vi "Variant To String.vi"(7 "Unsupported (Empty)":string, 10 "Variant":variant) -> (2 "Supported":bool, 3 "String":string)   [LabVIEW 2020, in "FlexBlocks.lvlib"]
uses:
  FlexBlocks.lvlib
  <vilib>/Utility/Data Type/NI_Data Type.lvlib
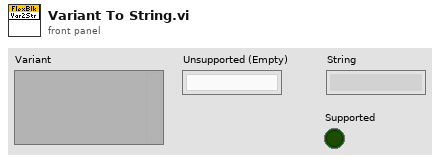
[diagram p1: front panel]
types:
  T1 = typedef "NI_Data Type.lvlib/Data Type.ctl" = enum8{"Invalid Type", "Void", "I8", "I16", "I32", "I64", "U8", "U16", "U32", "U64", "Single Float", "Double Float", "Extended Float", "Single Complex", "Double Complex", "Extended Complex", "Enum U8", "Enum U16", "Enum U32", "Enum U64", "Single Float With Unit", "Double Float With Unit", "Extended Float With Unit", "Single Complex with Unit", "Double Complex with Unit", "Extended Complex with Unit", "Boolean", "String", "Path", "Picture", "Tag", "Array", "Cluster", "Variant", "LV Variant", "Waveform", "Timestamp", "Digital Waveform", "Digital Data", "ExpressData", "Refnum", "External Data", "VI", "Poly VI", "LabVIEW Class Instance", "Fixed Point", "Set Collection", "Map Collection"}
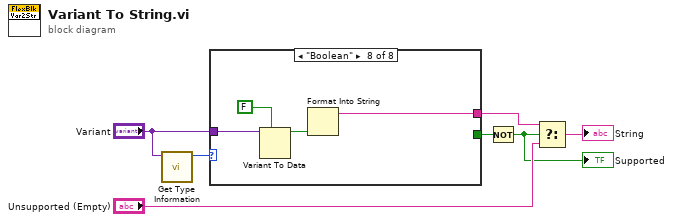
[diagram p0: block diagram]
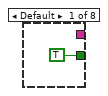
[diagram p2: hidden frame]
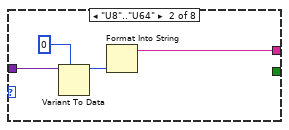
[diagram p3: hidden frame]
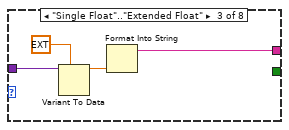
[diagram p4: hidden frame]
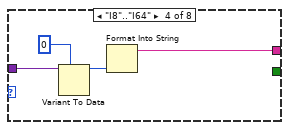
[diagram p5: hidden frame]
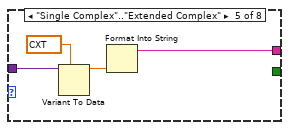
[diagram p6: hidden frame]
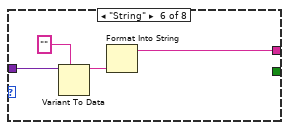
[diagram p7: hidden frame]
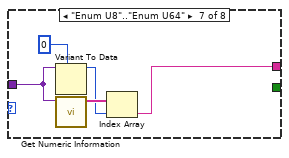
[diagram p8: hidden frame]
diagram:
  n1 = call <vilib>:"Get Type Information.vi"("variant"="Variant") -> ("type"=w5:T1)  [unwired: 6 in, 4 out]
  n2 = case shown="\"Boolean\"" w5 {
    tunnel: [TRUE _ _ _ _ _ _ _] -> w4
    tunnel: "Variant" -> [_ w12 w16 w20 w24 w28 w33 w37]
    tunnel: [_ w9 w13 w17 w21 w25 w29 w34] -> w1
    frame Default {
    }
    frame "U8".."U64" {
      n3 = Variant To Data(type=u64 0 ("U64"), Variant=w12) -> (data=w10:u64)  [unwired: 1 in, 1 out]
      n4 = Format Into String(w10) -> (resulting string=w9:string)  [unwired: 3 in, 1 out]
    }
    frame "Single Float".."Extended Float" {
      n5 = Variant To Data(type=ext 0.0 ("Ext"), Variant=w16) -> (data=w14:ext)  [unwired: 1 in, 1 out]
      n6 = Format Into String(w14) -> (resulting string=w13:string)  [unwired: 3 in, 1 out]
    }
    frame "I8".."I64" {
      n7 = Variant To Data(type=i64 0 ("I64"), Variant=w20) -> (data=w18:i64)  [unwired: 1 in, 1 out]
      n8 = Format Into String(w18) -> (resulting string=w17:string)  [unwired: 3 in, 1 out]
    }
    frame "Single Complex".."Extended Complex" {
      n9 = Variant To Data(type=cxt 0.0+0.0i ("I64"), Variant=w24) -> (data=w22:cxt)  [unwired: 1 in, 1 out]
      n10 = Format Into String(w22) -> (resulting string=w21:string)  [unwired: 3 in, 1 out]
    }
    frame "String" {
      n11 = Variant To Data(type="" ("I64"), Variant=w28) -> (data=w26:string)  [unwired: 1 in, 1 out]
      n12 = Format Into String(w26) -> (resulting string=w25:string)  [unwired: 3 in, 1 out]
    }
    frame "Enum U8".."Enum U64" {
      n13 = Variant To Data(type=u64 0, Variant=w33) -> (data=w30:u64)  [unwired: 1 in, 1 out]
      n14 = call <vilib>:"Get Numeric Information.vi"("variant"=w33) -> ("enum names"=w31:string[])  [unwired: 7 in, 3 out]
      n15 = Index Array(array=w31, index=w30) -> (element=w29:string)
    }
    frame "Boolean" {
      n16 = Variant To Data(type=FALSE, Variant=w37) -> (data=w35:bool)  [unwired: 1 in, 1 out]
      n17 = Format Into String(w35) -> (resulting string=w34:string)  [unwired: 3 in, 1 out]
    }
  }
  n18 = Not(x=w4) -> (.not. x?=w3:bool)
  "Supported" <- w3
  n19 = Select(t=w1, s=w3, f="Unsupported (Empty)") -> (s? t:f=→"String":string)
